vi "concatenate to radians.vi"(1 "value":dbl) -> (0 "concatenated value":dbl)   [LabVIEW 2009]
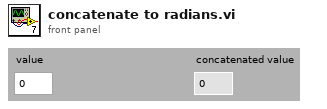
[diagram p1: front panel]
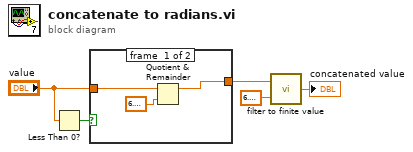
[diagram p0: block diagram]
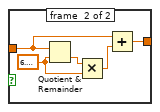
[diagram p2: hidden frame]
diagram:
  n1 = Less Than 0?(x="value") -> (x < 0?=w5:bool)
  n2 = case shown="True" w5 {
    tunnel: "value" -> [w8 w9]
    tunnel: [w6 w10] -> w2
    frame #0 {
      n3 = Quotient & Remainder(x=w8, y=6.283185307179586) -> (x-y*floor(x/y)=w6:dbl)  [unwired: 1 out]
    }
    frame #1 {
      w12 = 6.283185307179586
      n4 = Quotient & Remainder(x=w9, y=w12) -> (floor(x/y)=w13:dbl)  [unwired: 1 out]
      n5 = Multiply(x=w13, y=w12) -> (x*y=w11:dbl)
      n6 = Add(x=w9, y=w11) -> (x+y=w10:dbl)
    }
  }
  n7 = call "filter to finite value.vi"("replacement value"=6.283185307179586, "value"=w2) -> ("filtered value"=→"concatenated value":dbl)  [unwired: 1 in]
